vi "tsapp_get_lin_channel_count.vi"(8 "错误输入（无错误）":errorcluster, 11 "路径输入":path) -> (0 "错误输出":errorcluster, 1 "ACount":i32, 2 "return":i32, 3 "路径输出":path)   [LabVIEW 2014]
doc: "Function Introduction :\nGet the total number of LIN channels for the application\nCall location :\nAfter mapping the LIN channel, users can obtain the LIN channel according to the requirements of the application program\nquantity\ninput parameter :\nACount: Number of channels\nReturn value :\n==0: Execution successful\nOther values: Query error code"
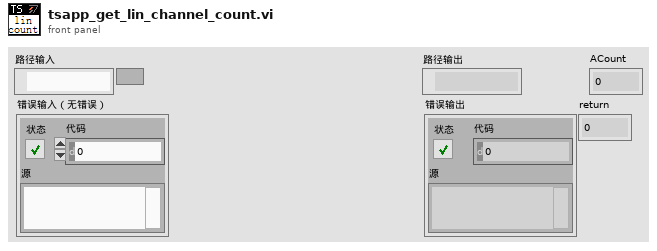
[diagram p1: front panel]
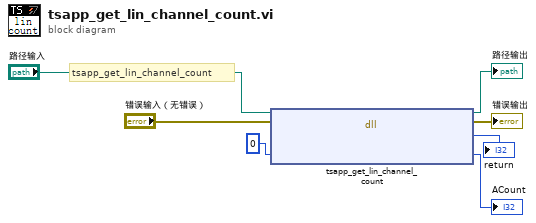
[diagram p0: block diagram]
diagram:
  # "tsapp_get_lin_channel_count"
  n1 = dll-call lib="D:/Program Files (x86)/TOSUN/TSMaster/Data/SDK/lib/x86/TSMaster.dll" fn="tsapp_get_lin_channel_count"(path in="路径输入", error in="错误输入（无错误）", "ACount"=0 ("Aount")) -> (path out=→"路径输出":path, error out=→"错误输出":errorcluster, "返回类型"=→"return":i32, "ACount"=→"ACount":i32)  [unwired: 1 in]
